vi "Stop Point.vi"(5 "Series Enqueuer":refnum<class "Message Enqueuer.lvclass">, 7 "Task-Point Ident":string, 8 "error in":errorcluster, 11 "MSS in":refnum<class "MSS.lvclass">) -> (0 "error out":errorcluster, 3 "MSS out":refnum<class "MSS.lvclass">)   [LabVIEW 2024, in "HAL.lvlib" / "MSS.lvclass"]
uses:
  MSS.lvclass
  <vilib>/ActorFramework/Message Enqueuer/Message Enqueuer.lvclass
  MSS.lvclass/MSS.ctl
  MAL/Series/ISeries Actor/ISeries Actor Messages/Log Event Msg/Log Event Msg.lvclass/Log Event Msg.ctl
  <vilib>/ActorFramework/Message Enqueuer/Message Enqueuer.lvclass/Message Enqueuer.ctl
  MAL/Series/ISeries Actor/ISeries Actor Messages/Stop Point on Target Msg/Stop Point on Target Msg.lvclass/Stop Point on Target Msg.ctl
  <vilib>/ActorFramework/Message Enqueuer/Enqueue.vi
  MAL/Series/ISeries Actor/ISeries Actor Messages/Log Event Msg/Log Event Msg.lvclass
  MAL/Series/ISeries Actor/ISeries Actor Messages/Stop Point on Target Msg/Stop Point on Target Msg.lvclass
  <vilib>/Utility/LVClass/Get LV Class Name.vi
  <resource>/AFDebug/Generate Trace for Message.vi
  <vilib>/ActorFramework/Message Priority Queue/Priority Enqueue.vi
  Virtual Instruments/Virtual Instrument/Virtual Instrument.lvclass
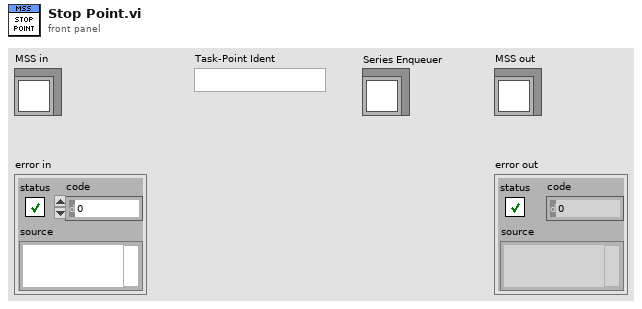
[diagram p1: front panel]
types:
  T1 = map{string, refnum<class "Virtual Instrument.lvclass">}
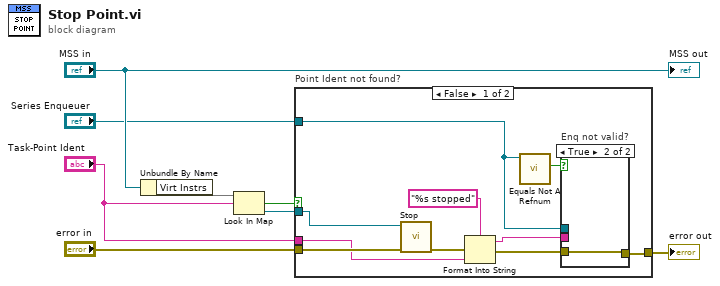
[diagram p0: block diagram]
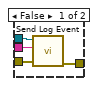
[diagram p2: hidden frame]
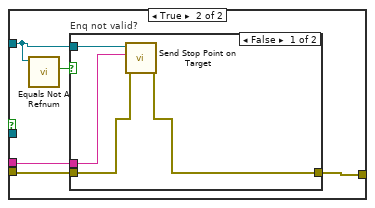
[diagram p3: hidden frame]
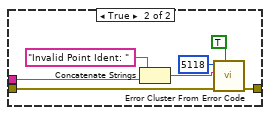
[diagram p4: hidden frame]
diagram:
  n1 = Unbundle By Name("MSS in") -> ("Virt Instrs"=w7:T1)
  n2 = Look In Map(map=w7, key="Task-Point Ident") -> (key not found?=w6:bool, value=w5:refnum<class "Virtual Instrument.lvclass">)  [unwired: 1 in]
  n3 = case "Point Ident not found?" shown="False" w6 {
    tunnel: w5 -> [w18 _]
    tunnel: "error in" -> [w17 w28]
    tunnel: [w12 w27] -> w4
    tunnel: "Series Enqueuer" -> [w10 w24]
    tunnel: "Task-Point Ident" -> [w9 w26]
    frame False {
      n4 = call "Stop.vi"("error in"=w17, "Virtual Instrument in"=w18) -> ("error out"=w14:errorcluster)  [unwired: 8 in, 1 out]
      n5 = Format Into String(format string="%s stopped", error in=w14, w9) -> (resulting string=w11:string, error out=w13:errorcluster)  [unwired: 1 in]
      n6 = call <vilib>:"Equals Not A Refnum.vi"("Message Enqueuer"=w10) -> ("Not a refnum?"=w15:bool)  [unwired: 10 in]
      n7 = case "Enq not valid?" shown="True" w15 {
        tunnel: w13 -> [w22 w23]
        tunnel: [w21 w23] -> w12
        tunnel: w11 -> [w20 _]
        tunnel: w10 -> [w19 _]
        frame False {
          n8 = call "Send Log Event.vi"("error in (no error)"=w22, "Event Text"=w20, "Message Enqueuer"=w19) -> ("error out"=w21:errorcluster)  [unwired: 7 in, 1 out]
        }
        frame True {
        }
      }
    }
    frame True {
      n9 = call <vilib>:"Equals Not A Refnum.vi"("Message Enqueuer"=w24) -> ("Not a refnum?"=w25:bool)  [unwired: 10 in]
      n10 = case "Enq not valid?" shown="False" w25 {
        tunnel: w28 -> [w30 w35]
        tunnel: [w29 w34] -> w27
        tunnel: w26 -> [w31 w33]
        tunnel: w24 -> [w32 _]
        frame False {
          n11 = call "Send Stop Point on Target.vi"("error in (no error)"=w30, "Point Ident"=w31, "Message Enqueuer"=w32) -> ("error out"=w29:errorcluster)  [unwired: 7 in, 1 out]
        }
        frame True {
          n12 = Concatenate Strings("Invalid Point Ident: ", w33) -> (w37:string)
          n13 = call <vilib>:"Error Cluster From Error Code.vi"("show call chain? (False)"=TRUE, "error in (no error)"=w35, "error message (\"\")"=w37, "error code (0)"=5118) -> ("error out"=w34:errorcluster)  [unwired: 5 in]
        }
      }
    }
  }
  "error out" <- w4
  "MSS out" <- "MSS in"
